vi "Read XML_Checks_Check Presence of labelOctal and labelDecimal.vi"(4 "labelOctalSpecified":bool, 6 "labelDecimalSpecified":bool, 7 "hardwareChannel":i32, 8 "error in (no error)":errorcluster, 10 "labelOctal":i32, 11 "labelDecimal":i32) -> (0 "error out":errorcluster, 3 "labelDecimal":i32)   [LabVIEW 2017]
doc: "This VI Checks whether either \"labelDecimal\" or \"labelOctal\" XML elements are present. There can only be one present. If none or 2, then an error -5017 is returned. The VI only returns first error detected."
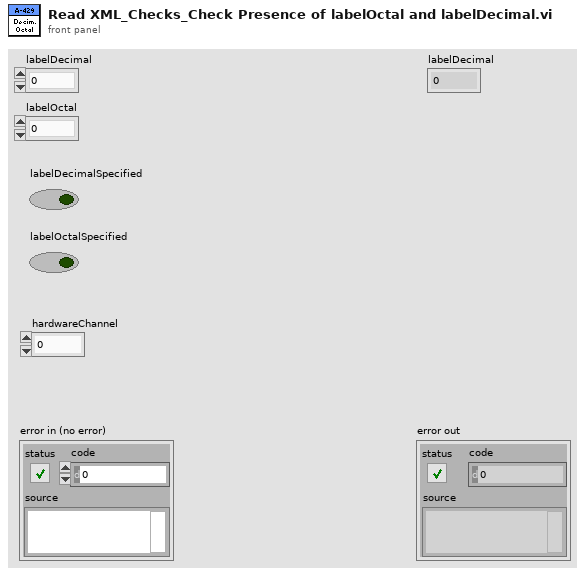
[diagram p1: front panel]
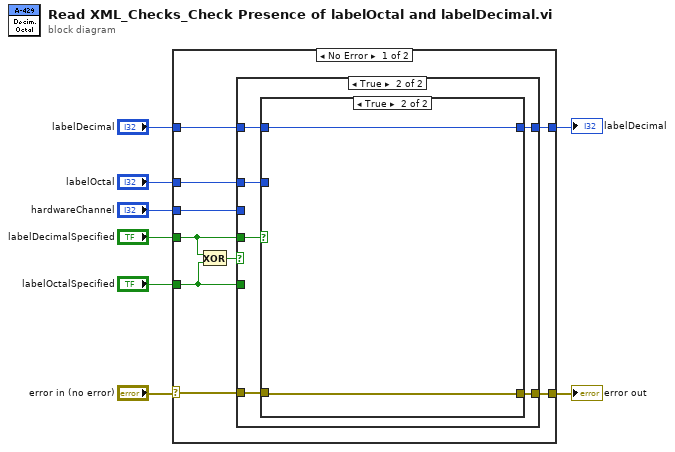
[diagram p0: block diagram]
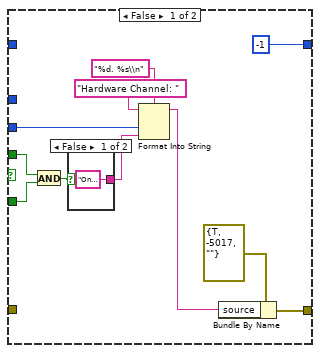
[diagram p2: hidden frame]
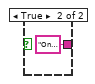
[diagram p3: hidden frame]
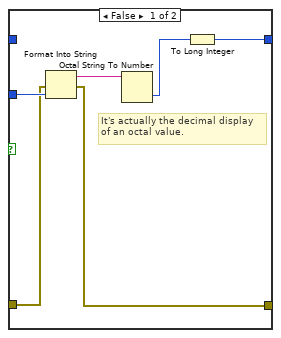
[diagram p4: hidden frame]
diagram:
  n1 = case shown="No Error" "error in (no error)" {
    selector: "error in (no error)" -> [w16 w46]
    tunnel: [w15 w46] -> w3
    tunnel: "labelDecimal" -> [w11 w45]
    tunnel: "labelOctal" -> [w10 _]
    tunnel: "labelDecimalSpecified" -> [w13 _]
    tunnel: "labelOctalSpecified" -> [w14 _]
    tunnel: "hardwareChannel" -> [w12 _]
    tunnel: [w9 w45] -> w1
    frame No Error {
      n2 = Exclusive Or(1:w14, 2:w13) -> (0:w17:bool)
      n3 = case shown="True" w17 {
        tunnel: w16 -> [_ w32]
        tunnel: [w28 w31] -> w15
        tunnel: w14 -> [w24 _]
        tunnel: w13 -> [w25 w36]
        tunnel: w12 -> [w22 _]
        tunnel: w11 -> [_ w35]
        tunnel: w10 -> [_ w33]
        tunnel: [-1 ("labelDecimal") w34] -> w9
        frame False {
          n4 = And(x=w25, y=w24) -> (x .and. y?=w21:bool)
          n5 = case shown="False" w21 {
            tunnel: ["One (but only one) of the \"labelOctal\" and \"labelDecimal\" XML elements must be present for a given Label." "Only one of the \"labelOctal\" and \"labelDecimal\" XML elements can be present for a given Label."] -> w20
            frame False {
            }
            frame True {
            }
          }
          n6 = Format Into String(format string="%d. %s\\n", initial string="Hardware Channel: ", w22, w20) -> (resulting string=w26:string)  [unwired: 1 in, 1 out]
          n7 = Bundle By Name(cluster=errorcluster {"status"=TRUE, "code"=-5017, "source"=""} ("error IO"), "source"=w26) -> (w28:errorcluster)
        }
        frame True {
          n8 = case shown="True" w36 {
            tunnel: w35 -> [_ w44]
            tunnel: [w37 w44] -> w34
            tunnel: w33 -> [w42 _]
            tunnel: w32 -> [w41 w43]
            tunnel: [w40 w43] -> w31
            frame False {
              # "It's actually the decimal display\nof an octal value."
              n9 = Format Into String(error in=w41, w42) -> (resulting string=w39:string, error out=w40:errorcluster)  [unwired: 2 in]
              n10 = Octal String To Number(4:w39) -> (0:w38:u32)  [unwired: 2 in, 1 out]
              n11 = To Long Integer(number=w38) -> (32bit integer=w37:i32)
            }
            frame True {
            }
          }
        }
      }
    }
    frame Error {
    }
  }
  "error out" <- w3
  "labelDecimal" <- w1
